vi "set speed.vi"(0 "VISA resource name":refnum<visa-resource-name>, 1 "Device Number":i8, 2 "Speed":i32, 3 "error in (no error)":errorcluster) -> (5 "VISA resource name out":refnum<visa-resource-name>, 6 "error out":errorcluster)   [LabVIEW 2020]
uses:
  ZaberTSeries.lvlib
panel:
  in  "Reponse Count":i32=1
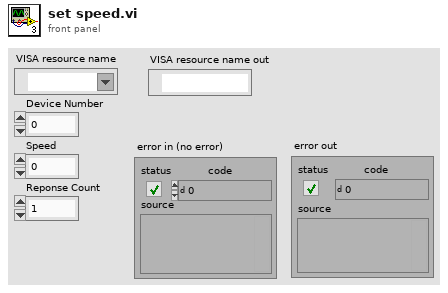
[diagram p1: front panel]
types:
  T1 = cluster{"Device Number":i8, "Command for setting speed":i8, "Speed":i32, "Reponse Count":i32}
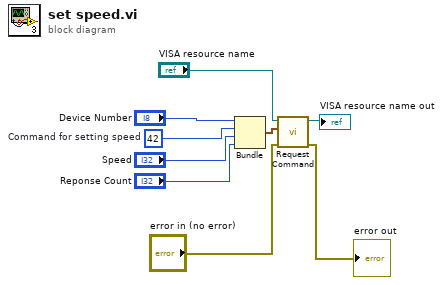
[diagram p0: block diagram]
diagram:
  w6 = i8 42  # Command for setting speed
  n1 = Bundle("Device Number"="Device Number", "Command for setting speed"=w6, "Speed"="Speed", "Reponse Count"="Reponse Count") -> (w3:T1)  [unwired: 1 in]
  n2 = call "Request Command.vi"("error in (no error)"="error in (no error)", "Request"=w3, "VISA resource name"="VISA resource name") -> ("error out"=→"error out":errorcluster, "VISA resource name out"=→"VISA resource name out":refnum<visa-resource-name>)  [unwired: 5 in, 2 out]
